vi "Refresh User.vi"(8 "error in (no error)":errorcluster, 10 "User In":refnum<class "User.lvclass">, 11 "User Provider in":refnum<class "User Provider.lvclass">) -> (0 "error out":errorcluster, 2 "User":refnum<class "User.lvclass">, 3 "User Provider out":refnum<class "User Provider.lvclass">)   [LabVIEW 2022 SP3, in "HTTP-Conditum.lvlib" / "User Provider.lvclass"]
uses:
  User Provider.lvclass
  <vilib>/IlluminatedG/IG HTTP Server/HTTP Server/User/User.lvclass
  User Provider.lvclass/User Provider.ctl
  <vilib>/IlluminatedG/IG Conditum/Conditum/Entity Manager/Entity Manager.lvclass
  User/User.lvclass
  C:/Program Files (x86)/National Instruments/LabVIEW 2022/vi.lib/IlluminatedG/IG Conditum/Conditum/Entity/Entity.lvclass
  C:/Program Files (x86)/National Instruments/LabVIEW 2022/vi.lib/IlluminatedG/IG HTTP Server/HTTP Server/User/User.lvclass
  C:/Program Files (x86)/National Instruments/LabVIEW 2022/vi.lib/IlluminatedG/IG HTTP Server/HTTP Server/Service/Service.lvclass
  C:/dev/lv/illuminated-g/lv-http-conditum/HTTP-Conditum/User/User.lvclass
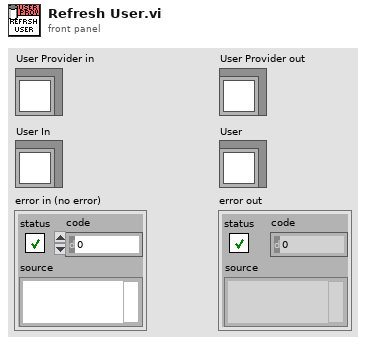
[diagram p1: front panel]
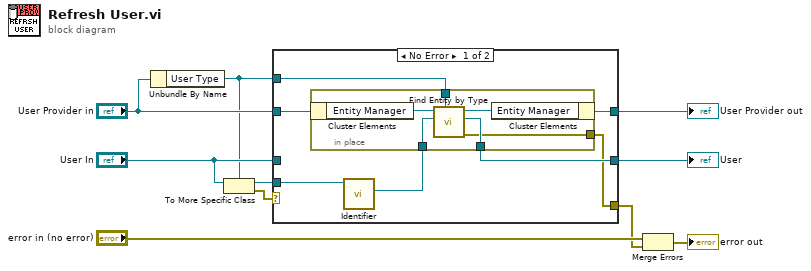
[diagram p0: block diagram]
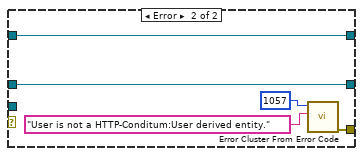
[diagram p2: hidden frame]
diagram:
  n1 = Unbundle By Name("User Provider in") -> ("User Type"=w1:refnum<class "User.lvclass">)
  n2 = To More Specific Class(target class=w1, reference="User In") -> (specific class reference=w9:refnum<class "User.lvclass">, error out=w5:errorcluster)  [unwired: 1 in]
  n3 = case shown="No Error" w5 {
    tunnel: w9 -> [w16 _]
    tunnel: [w15 w27] -> w8
    tunnel: "User Provider in" -> [w12 w26]
    tunnel: [w14 w26] -> w7
    tunnel: "User In" -> [_ w27]
    tunnel: [w13 w28] -> w3
    tunnel: w1 -> [w11 _]
    frame No Error {
      n4 = call "Identifier.vi"("User in"=w16) -> ("Identifier"=w17:refnum<class "Type.lvclass">)  [unwired: 10 in]
      n5 = in-place {
        in-place-border: w17 -> [w23]
        in-place-border: [w22] -> w15
        in-place-border: [w19] -> w13
        in-place-border: w11 -> [w18]
        n6 = in-place-cluster #1(w12) -> ("Entity Manager"=w21:refnum<class "Entity Manager.lvclass">)
        n7 = call <vilib>:"Find Entity by Type.vi"("Entity Type"=w18, "Type"=w23, "Entity Manager in"=w21) -> ("error out"=w19:errorcluster, "Entity"=w22:refnum<class "User.lvclass">, "Entity Manager out"=w20:refnum<class "Entity Manager.lvclass">)  [unwired: 6 in]
        n8 = in-place-cluster #1("Entity Manager"=w20) -> (w14:refnum<class "User Provider.lvclass">)
      }
    }
    frame Error {
      n9 = call <vilib>:"Error Cluster From Error Code.vi"("error message (\"\")"="User is not a HTTP-Conditum:User derived entity." ("error message (\"\")"), "error code (0)"=1057) -> ("error out"=w28:errorcluster)  [unwired: 7 in]
    }
  }
  "User Provider out" <- w7
  "User" <- w8
  n10 = Merge Errors("error in (no error)", w3) -> (→"error out":errorcluster)
